vi "SQL_Fetch All Data.vi"(8 "error in (no error)":errorcluster, 9 "MCListBox":refnum<vi>, 10 "Table":string, 11 "SQL in":refnum<class "SQL.lvclass">) -> (0 "error out":errorcluster, 1 "columns":string[](array[string]), 2 "InitialData":string[][](array[string]), 3 "SQL out":refnum<class "SQL.lvclass">)   [LabVIEW 2012, in "SQL.lvclass"]
uses:
  SQL.lvclass
  <vilib>/addons/database/_DB Variant To Data/Database Variant To Data.xnode
  <vilib>/addons/database/NI_Database_API.lvlib
panel:
  out "MCListBox":refnum<vi>
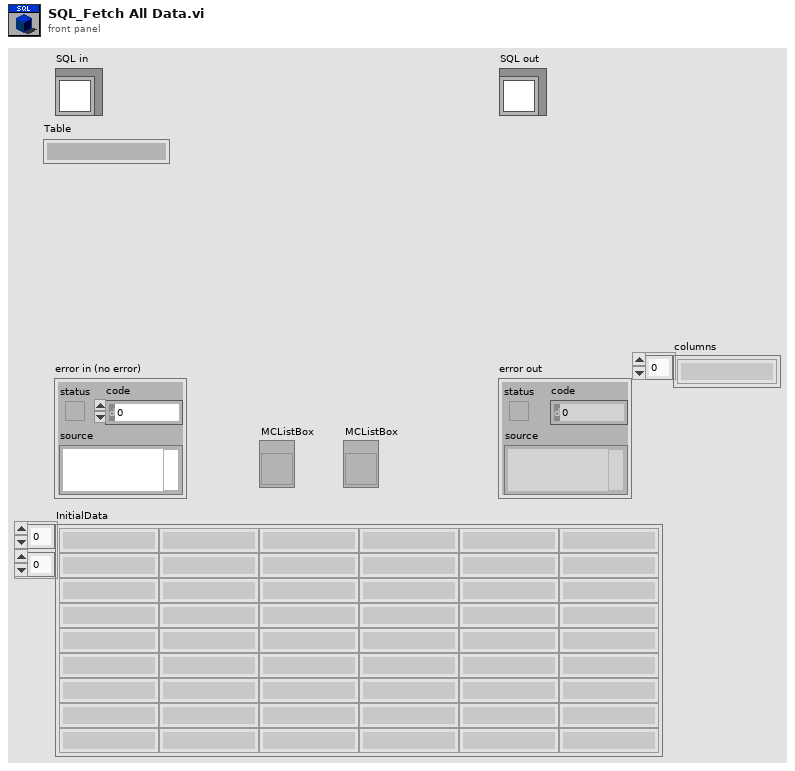
[diagram p1: front panel]
types:
  T1 = typedef "SQL.lvclass/ObjectAttributes.ctl" = cluster{"DB Connection Reference":T2}
  T2 = typedef "NI_Database_API.lvlib/Conn ObjectReference.ctl" = refnum<k1>
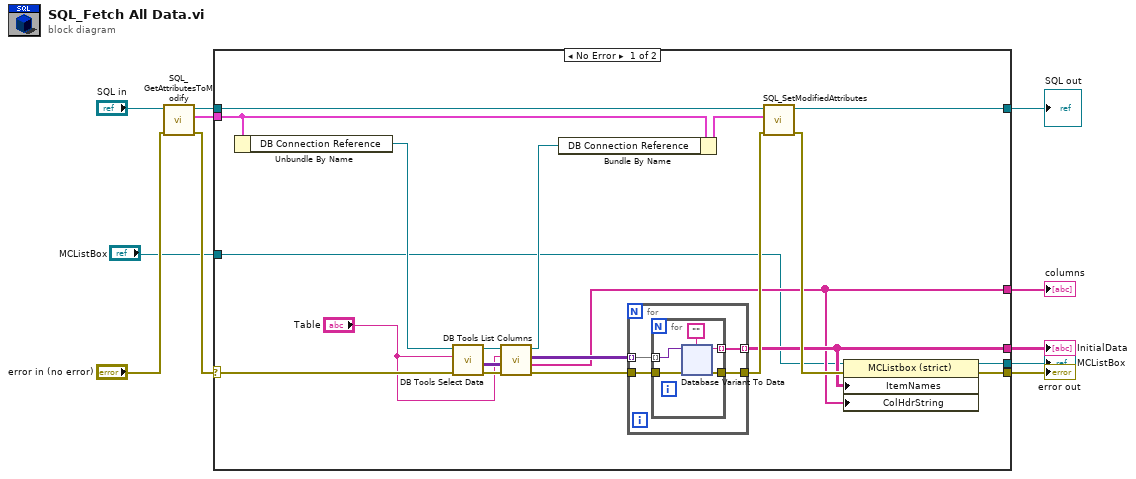
[diagram p0: block diagram]
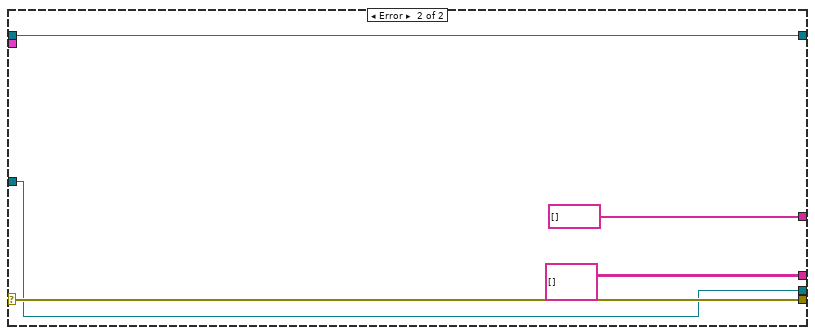
[diagram p2: hidden frame]
diagram:
  n1 = call "SQL_GetAttributesToModify.vi"("error in (no error)"="error in (no error)", "reference in"="SQL in") -> ("error out"=w4:errorcluster, "Attributes"=w7:T1, "reference out"=w8:refnum<class "SQL.lvclass">)  [unwired: 6 in, 1 out]
  n2 = case shown="No Error" w4 {
    selector: w4 -> [w27 w76]
    tunnel: [w16 w76] -> w11
    tunnel: [w29 w75] -> w10
    tunnel: w8 -> [w30 w75]
    tunnel: w7 -> [w26 _]
    tunnel: [w15 string[][] []] -> w6
    tunnel: [w14 string[] [] ("columns")] -> w3
    tunnel: [w13 w72] -> w2
    tunnel: "MCListBox" -> [w12 w72]
    frame No Error {
      n3 = Unbundle By Name(w26) -> ("DB Connection Reference"=w24:T2)
      n4 = call <vilib>:"DB Tools Select Data.vi"("error in (no error)"=w27, "table"="Table", "connection reference"=w24) -> ("error out"=w22:errorcluster, "data"=w28:variant[][], "connection reference out"=w20:T2)  [unwired: 3 in]
      n5 = call <vilib>:"DB Tools List Columns.vi"("error in (no error)"=w22, "table"="Table", "connection reference"=w20) -> ("error out"=w21:errorcluster, "columns"=w14:string[], "connection reference out"=w18:T2)  [unwired: 1 in, 1 out]
      n6 = Bundle By Name(cluster=w26, "DB Connection Reference"=w18) -> (w25:T1)
      n7 = for {
        tunnel: w28 -> [w34] mode=indexing
        tunnel: [w33] -> w15 mode=indexing
        tunnel: [w32] -> w23
        tunnel: w21 -> [w31]
        n8 = for {
          tunnel: w34 -> [w38] mode=indexing
          tunnel: [w37] -> w33 mode=indexing
          tunnel: [w36] -> w32
          tunnel: w31 -> [w35]
          n9 = xnode "Database Variant To Data"("database variant"=w38, "error in"=w35, "type"="") -> ("data"=w37:string, "error out"=w36:errorcluster)
        }
      }
      n10 = call "SQL_SetModifiedAttributes.vi"("error in (no error)"=w23, "Attributes"=w25, "reference in"=w30) -> ("error out"=w17:errorcluster, "reference out"=w29:refnum<class "SQL.lvclass">)  [unwired: 7 in]
      n11 = property on="Property Node" class="MCListbox (strict)"(reference=w12, error in=w17, "ItemNames"=w15, "ColHdrString"=w14) -> (reference out=w13:refnum<vi>, error out=w16:errorcluster)
    }
    frame Error {
    }
  }
  "error out" <- w11
  "SQL out" <- w10
  "InitialData" <- w6
  "columns" <- w3
  "MCListBox" <- w2
